vi "Set Current Caster Angle.vi"(8 "error in (no error)":errorcluster, 10 "current caster angle (rad)":dbl, 11 "caster wheel in":refnum<class "NI_Robotics_Caster Wheel.lvclass">) -> (0 "error out":errorcluster, 3 "caster wheel out":refnum<class "NI_Robotics_Caster Wheel.lvclass">)   [LabVIEW 2017, in "NI_Robotics_Caster Wheel.lvclass"]
uses:
  <vilib>/robotics/Steering/Caster Wheel/NI_Robotics_Caster Wheel.lvclass
  <vilib>/robotics/Steering/Caster Wheel/NI_Robotics_Caster Wheel.lvclass/NI_Robotics_Caster Wheel.ctl
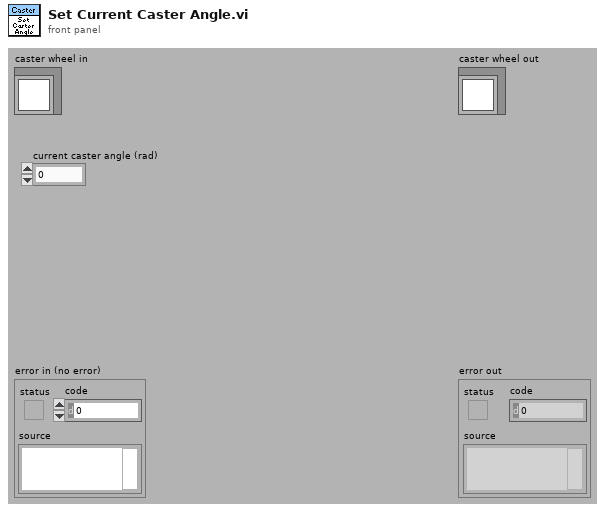
[diagram p1: front panel]
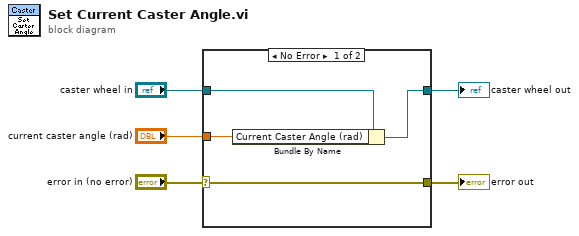
[diagram p0: block diagram]
diagram:
  n1 = case shown="No Error" "error in (no error)" {
    selector: "error in (no error)" -> [w6 w10]
    tunnel: "current caster angle (rad)" -> [w8 _]
    tunnel: "caster wheel in" -> [w9 w11]
    tunnel: [w7 w11] -> w2
    tunnel: [w6 w10] -> w1
    frame No Error {
      n2 = Bundle By Name(cluster=w9, "Current Caster Angle (rad)"=w8) -> (w7:refnum<class "NI_Robotics_Caster Wheel.lvclass">)
    }
    frame Error {
    }
  }
  "error out" <- w1
  "caster wheel out" <- w2
